vi "Check Disk Space.vi"(8 "Error In":errorcluster, 11 "Frame Grabber Data":T1={"Camera Session"="", "Frame"=refnum, "AVI Refnum"=refnum, "Codecs"=[], "Frame number"=0, "Tracking File Refnum"=refnum, "Tick Count"=0, "Probe Object"=refnum, "Playback Probe Data"=[], "Rigid Body"={"Position"={"x (mm)"=0.0, "y (mm)"=0.0, "z (mm)"=0.0}, "Orientation"={"Pitch (rad)"=0.0, "Yaw (rad)"=0.0, "Roll (rad)"=0.0}, "Quaternion"={"qx"=0.0, "qy"=0.0, "qz"=0.0, "qw"=0.0}, "Tracked?"=FALSE}, "Total no frames playback"=0, "Video FPS"=0.0, "Camera connected?"=FALSE, "Scene"=refnum, "Cropped Frame"=refnum, "Tracker FPS"=0.0, "Crop ROI"=[], "Presentation Values"=[], "Elapsed time (ms)"=0, "Camera frames playback"=0, "Refnums"={"Live Refnum"=refnum, "Record Refnum"=refnum, "Recording Settings Refnum"=refnum, "Playback Refnum"=refnum, "Frame Slider Refnum"=refnum, "Pause Refnum"=refnum, "Home Refnum"=refnum, "Crop Refnum"=refnum, "Clear Crop Refnum"=refnum, "stop refnum"=refnum, "Playback Rate Refnum"=refnum, "Operator Settings Refnums"=refnum, "Presentation Refnum"=refnum, "Gestation Refnum"=refnum, "Connection Settings Refnum"=refnum, "Crop Time Frame Slider Refnum"=refnum, "Cancel Save Refnum"=refnum}, "Dimensions"={"Probe Dimensions"={"Probe Width"=0.0, "Probe Depth"=1.0, "Probe Height"=0.0}, "Room Dimensions"={"Room Width"=0.0, "Room Depth"=0.0, "Room Height"=0.0}}, "Playback Data As Strings"=[], "Cropped Tracking File Refnum"=refnum, "Cropped AVI Refnum"=refnum, "Header"=[]}) -> (0 "Error Out":errorcluster, 1 "free (bytes)":i64, 2 "Max number of frames":dbl, 3 "Prompt":string, 4 "Size per frame (bytes)":dbl)   [LabVIEW 2017]
uses:
  Controls/Frame Grabber Data.ctl
  <vilib>/userdefined/High Color/IMAQdx.ctl
  <vilib>/vision/Image Controls.llb/IMAQ Image.ctl
  <vilib>/vision/Avi.llb/IMAQ AVI2 Refnum.ctl
  Controls/Rigid Body Info.ctl
  Controls/Position.ctl
  Controls/Orientation.ctl
  Controls/Refnums.ctl
  Controls/Recording Settings.ctl
  Controls/Operator Settings.ctl
  Controls/Operator.ctl
  Controls/Dimensions.ctl
  Controls/Room Dimensions.ctl
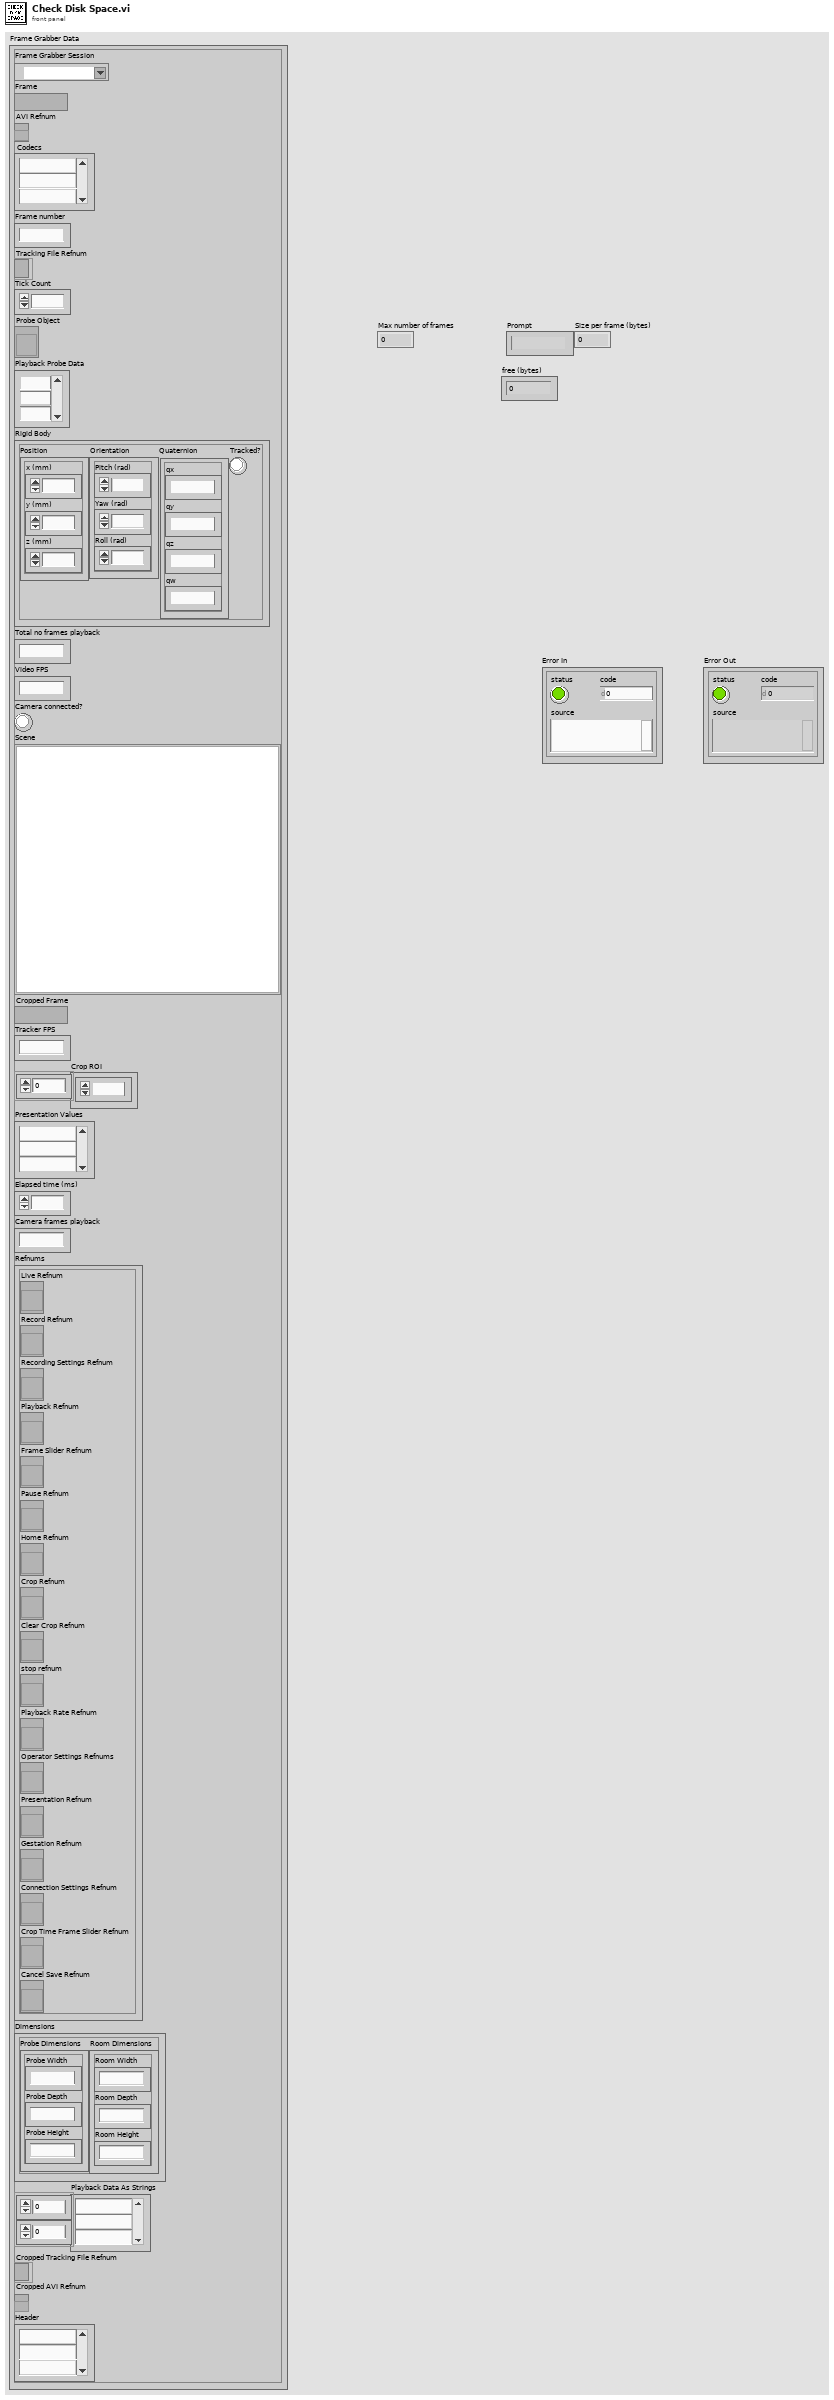
[diagram p1: front panel]
types:
  T1 = typedef "Frame Grabber Data.ctl" = cluster{"Camera Session":T2, "Frame":T3, "AVI Refnum":T4, "Codecs":string[], "Frame number":u32, "Tracking File Refnum":refnum<file>, "Tick Count":u32, "Probe Object":refnum<vi>, "Playback Probe Data":dbl[][], "Rigid Body":T5, "Total no frames playback":i32, "Video FPS":dbl, "Camera connected?":bool, "Scene":refnum<vi>, "Cropped Frame":T3, "Tracker FPS":dbl, "Crop ROI":i32[], "Presentation Values":string[], "Elapsed time (ms)":u32, "Camera frames playback":u32, "Refnums":T8, "Dimensions":T9, "Playback Data As Strings":string[][], "Cropped Tracking File Refnum":refnum<file>, "Cropped AVI Refnum":T4, "Header":string[]}
  T2 = typedef "IMAQdx.ctl" = refnum<k21>
  T3 = typedef "IMAQ Image.ctl" = refnum<image>
  T4 = typedef "IMAQ AVI2 Refnum.ctl" = refnum<k20>
  T5 = typedef "Rigid Body Info.ctl" = cluster{"Position":T6, "Orientation":T7, "Quaternion":cluster{"qx":sgl, "qy":sgl, "qz":sgl, "qw":sgl}, "Tracked?":bool}
  T6 = typedef "Position.ctl" = cluster{"x (mm)":sgl, "y (mm)":sgl, "z (mm)":sgl}
  T7 = typedef "Orientation.ctl" = cluster{"Pitch (rad)":sgl, "Yaw (rad)":sgl, "Roll (rad)":sgl}
  T8 = typedef "Refnums.ctl" = cluster{"Live Refnum":refnum<vi>, "Record Refnum":refnum<vi>, "Recording Settings Refnum":refnum<vi>, "Playback Refnum":refnum<vi>, "Frame Slider Refnum":refnum<vi>, "Pause Refnum":refnum<vi>, "Home Refnum":refnum<vi>, "Crop Refnum":refnum<vi>, "Clear Crop Refnum":refnum<vi>, "stop refnum":refnum<vi>, "Playback Rate Refnum":refnum<vi>, "Operator Settings Refnums":refnum<vi>, "Presentation Refnum":refnum<vi>, "Gestation Refnum":refnum<vi>, "Connection Settings Refnum":refnum<vi>, "Crop Time Frame Slider Refnum":refnum<vi>, "Cancel Save Refnum":refnum<vi>}
  T9 = typedef "Dimensions.ctl" = cluster{"Probe Dimensions":cluster{"Probe Width":sgl, "Probe Depth":sgl, "Probe Height":sgl}, "Room Dimensions":T10}
  T10 = typedef "Room Dimensions.ctl" = cluster{"Room Width":dbl, "Room Depth":dbl, "Room Height":dbl}
  T11 = typedef "Recording Settings.ctl" = cluster{"Folder to Save Recording":path, "Recording Name":string, "Video FPS":dbl, "Codec":u16, "Tracker FPS":dbl}
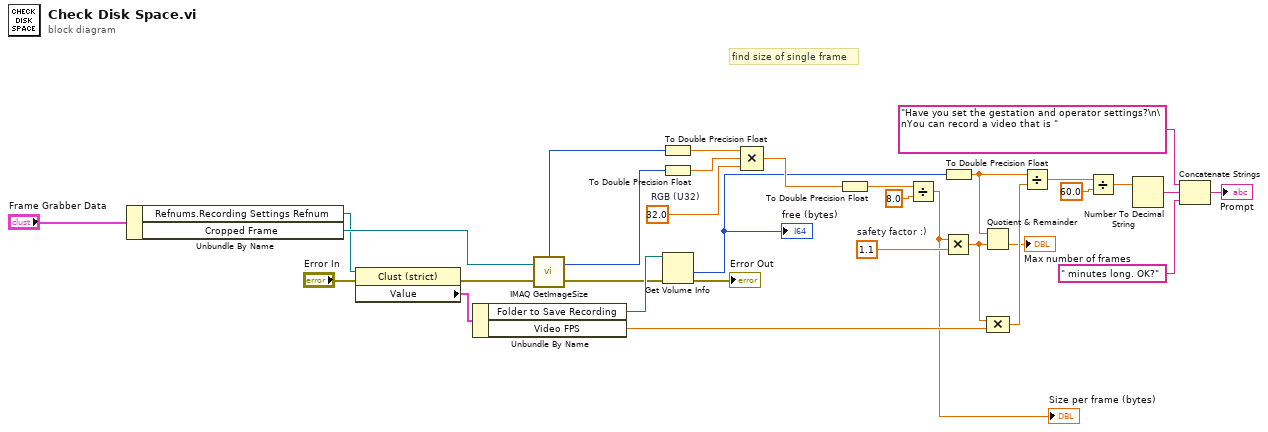
[diagram p0: block diagram]
diagram:
  w12 = 1.1  # safety factor :)
  w28 = 32.0  # RGB (U32)
  # "find size of single frame"
  n1 = Unbundle By Name("Frame Grabber Data") -> ("Refnums.Recording Settings Refnum"=w4:refnum<vi>, "Cropped Frame"=w8:T3)
  n2 = property class="Clust (strict)"(reference=w4, error in="Error In") -> (error out=w1:errorcluster, "Value"=w3:T11)  [unwired: 1 out]
  n3 = Unbundle By Name(w3) -> ("Folder to Save Recording"=w25:path, "Video FPS"=w23:dbl)
  n4 = call "IMAQ GetImageSize"("Image"=w8, "error in (no error)"=w1) -> ("Y Resolution"=w7:i32, "X Resolution"=w6:i32, "error out"=w5:errorcluster)  [unwired: 2 in]
  n5 = To Double Precision Float(number=w6) -> (double precision float=w27:dbl)
  n6 = To Double Precision Float(number=w7) -> (double precision float=w26:dbl)
  n7 = Get Volume Info(8:w5, 11:w25) -> (0:→"Error Out":errorcluster, 1:w22:i64)  [unwired: 4 out]
  "free (bytes)" <- w22
  n8 = Compound Arithmetic op=MULTIPLY(w27, w26, w28) -> (w30:dbl)
  n9 = To Double Precision Float(number=w30) -> (double precision float=w29:dbl)
  n10 = Divide(x=w29, y=8.0) -> (x/y=w11:dbl)
  "Size per frame (bytes)" <- w11
  n11 = Multiply(x=w11, y=w12) -> (x*y=w10:dbl)
  n12 = To Double Precision Float(number=w22) -> (double precision float=w13:dbl)
  n13 = Quotient & Remainder(x=w13, y=w10) -> (floor(x/y)=→"Max number of frames":dbl)  [unwired: 1 out]
  n14 = Compound Arithmetic op=MULTIPLY(w10, w23) -> (w21:dbl)
  n15 = Divide(x=w13, y=w21) -> (x/y=w20:dbl)
  n16 = Divide(x=w20, y=60.0) -> (x/y=w18:dbl)
  n17 = Number To Decimal String(number=w18) -> (decimal integer string=w17:string)  [unwired: 1 in]
  n18 = Concatenate Strings("Have you set the gestation and operator settings?\n\nYou can record a video that is " ("string"), w17, " minutes long. OK?" ("string")) -> (→"Prompt":string)
